vi "Check STFT Params.vi"(8 "compare signal and window?":bool=TRUE, 9 "windows length":i32, 10 "time increment":i32, 11 "len(X)":i32) -> (0 "error":i32, 3 "time step out":i32)   [LabVIEW 2010, in "NI_Gmath.lvlib"]
uses:
  NI_Gmath.lvlib
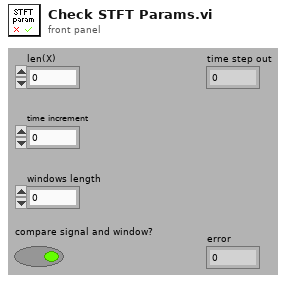
[diagram p1: front panel]
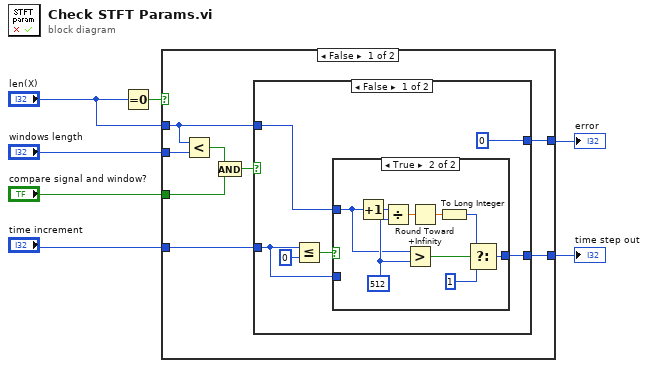
[diagram p0: block diagram]
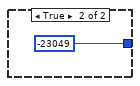
[diagram p3: hidden frame]
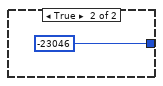
[diagram p4: hidden frame]
diagram:
  n1 = Equal To 0?(x="len(X)") -> (x = 0?=w4:bool)
  n2 = case shown="False" w4 {
    tunnel: [w14 -23046] -> w5
    tunnel: "windows length" -> [w15 _]
    tunnel: "len(X)" -> [w13 _]
    tunnel: "time increment" -> [w12 _]
    tunnel: [w11 _] -> w2
    tunnel: "compare signal and window?" -> [w9 _]
    frame False {
      n3 = Less?(x=w13, y=w15) -> (x < y?=w10:bool)
      n4 = And(x=w10, y=w9) -> (x .and. y?=w8:bool)
      n5 = case shown="False" w8 {
        tunnel: [0 -23049] -> w14
        tunnel: w13 -> [w20 _]
        tunnel: w12 -> [w18 _]
        tunnel: [w16 _] -> w11
        frame False {
          n6 = Less Or Equal?(x=w18, y=0) -> (x <= y?=w17:bool)
          n7 = case shown="True" w17 {
            tunnel: [w22 w29] -> w16
            tunnel: w18 -> [w22 _]
            tunnel: w20 -> [_ w24]
            frame False {
            }
            frame True {
              w28 = 512 ("y")
              n8 = Increment(x=w24) -> (x+1=w23:i32)
              n9 = Divide(x=w23, y=w28) -> (x/y=w27:dbl)
              n10 = Greater?(x=w24, y=w28) -> (0:w31:bool)
              n11 = Round Toward +Infinity(x=w27) -> (ceil(x): smallest int >= x=w26:dbl)
              n12 = To Long Integer(number=w26) -> (32bit integer=w25:i32)
              n13 = Select(t=w25, s=w31, f=1) -> (s? t:f=w29:i32)
            }
          }
        }
        frame True {
        }
      }
    }
    frame True {
    }
  }
  "error" <- w5
  "time step out" <- w2
